vi "scaleIMU.vi"(1 "Gyro Scale":enum16{"250dps", "500dps", "1000dps", "2000dps"}(ring), 2 "Accel Scale":enum16{"2g", "4g", "8g", "16g"}(ring), 3 "SPI Config In":T1) -> (0 "SPI Config Out":T1)   [LabVIEW 2019]
uses:
  SPI/SPI Config.ctl
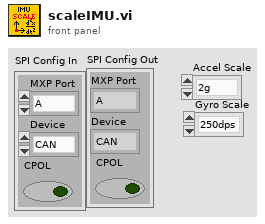
[diagram p1: front panel]
types:
  T1 = typedef "SPI Config.ctl" = cluster{"MXP Port":enum16{"A", "B"}, "Device":enum16{"CAN", "ENC", "IMU1", "IMU2"}, "CPOL":bool}
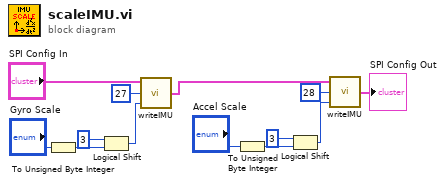
[diagram p0: block diagram]
diagram:
  n1 = To Unsigned Byte Integer(number="Gyro Scale") -> (unsigned 8bit integer=w12:u8)
  n2 = Logical Shift(y=i16 3, x=w12) -> (x << y=w10:u8)
  n3 = call "writeIMU.vi"("Data"=w10, "Address"=u8 27, "SPI Config In"="SPI Config In") -> ("SPI Config Out"=w8:T1)
  n4 = To Unsigned Byte Integer(number="Accel Scale") -> (unsigned 8bit integer=w7:u8)
  n5 = Logical Shift(y=i16 3, x=w7) -> (x << y=w4:u8)
  n6 = call "writeIMU.vi"("Data"=w4, "Address"=u8 28, "SPI Config In"=w8) -> ("SPI Config Out"=→"SPI Config Out":T1)
